vi "manual intake logic.vi"(9 "cone cube stuff":T1, 10 "intake modes":T2, 11 "grid-dy":T3(array[cluster])=[{"cascade pos"=12.0, "wrist pos"=30.0, "roller pow"=0.8}]) -> (2 "new object":T1, 3 "sign convention value":dbl)   [LabVIEW 2020]
uses:
  manipulator/Implementation/Typedefs/game object.ctl
  Typedef/intake typedef.ctl
  manipulator/Implementation/Typedefs/the grid-dy.ctl
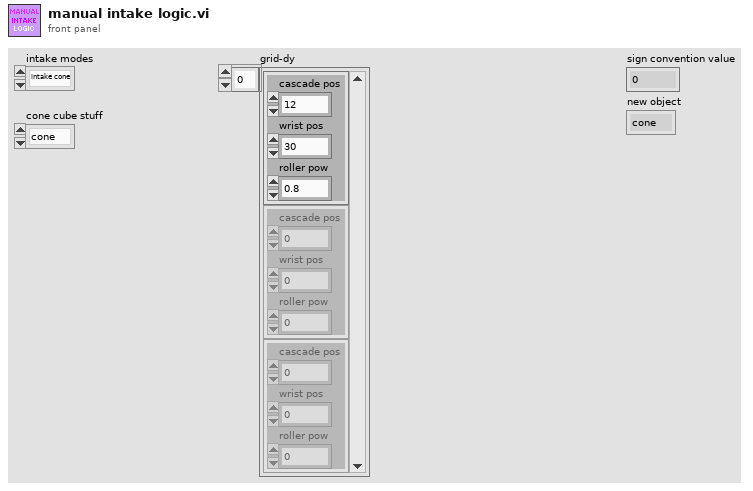
[diagram p1: front panel]
types:
  T1 = typedef "game object.ctl" = enum16{"cone", "cube"}
  T2 = typedef "intake typedef.ctl" = enum16{"intake cone", "intake cube", "outtake cone", "outtake cube"}
  T3 = cluster{"cascade pos":dbl, "wrist pos":dbl, "roller pow":dbl}[]
  T4 = typedef "the grid-dy.ctl" = enum16{"idle", "intake cone", "intake cube", "score low cone outtake", "score low cube outtake", "score mid cone", "score mid cube", "score high cone", "score high cube"}
  T5 = cluster{"cascade pos":dbl, "wrist pos":dbl, "roller pow":dbl}
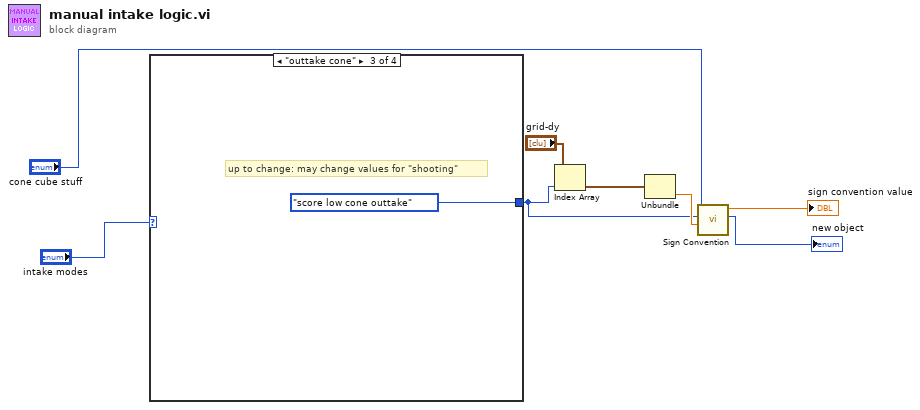
[diagram p0: block diagram]
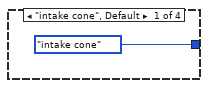
[diagram p2: hidden frame]
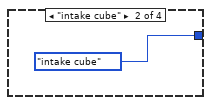
[diagram p3: hidden frame]
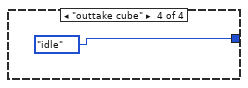
[diagram p4: hidden frame]
diagram:
  n1 = case shown="\"outtake cone\"" "intake modes" {
    tunnel: [the_grid-dy."intake cone" ("Enum") the_grid-dy."intake cube" ("Enum") the_grid-dy."score low cone outtake" ("Enum") the_grid-dy."idle" ("Enum")] -> w3
    frame "intake cone", Default {
    }
    frame "intake cube" {
    }
    frame "outtake cone" {
      # "up to change: may change values for \"shooting\""
    }
    frame "outtake cube" {
    }
  }
  n2 = Index Array(array="grid-dy", index=w3) -> (element=w6:T5)
  n3 = Unbundle(w6) -> ("roller pow"=w5:dbl)  [unwired: 2 out]
  n4 = call "Sign Convention.vi"("intake speed"=w5, "grid-dy commands"=w3, "current object"="cone cube stuff") -> ("new object"=→"new object":T1, "sign convention value"=→"sign convention value":dbl)  [unwired: 7 in]
